vi "Test@ShowCMD__Parameter.vi"(1 "ParamterIn":string) -> (0 "ParamterOut":string)   [LabVIEW 2019]
panel:
  in  "Device":string(combo)
  in  "Confirm":bool
  # "Test@ShowCMD $ExternDevice"
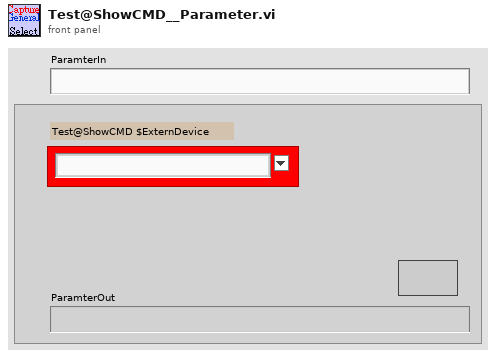
[diagram p1: front panel]
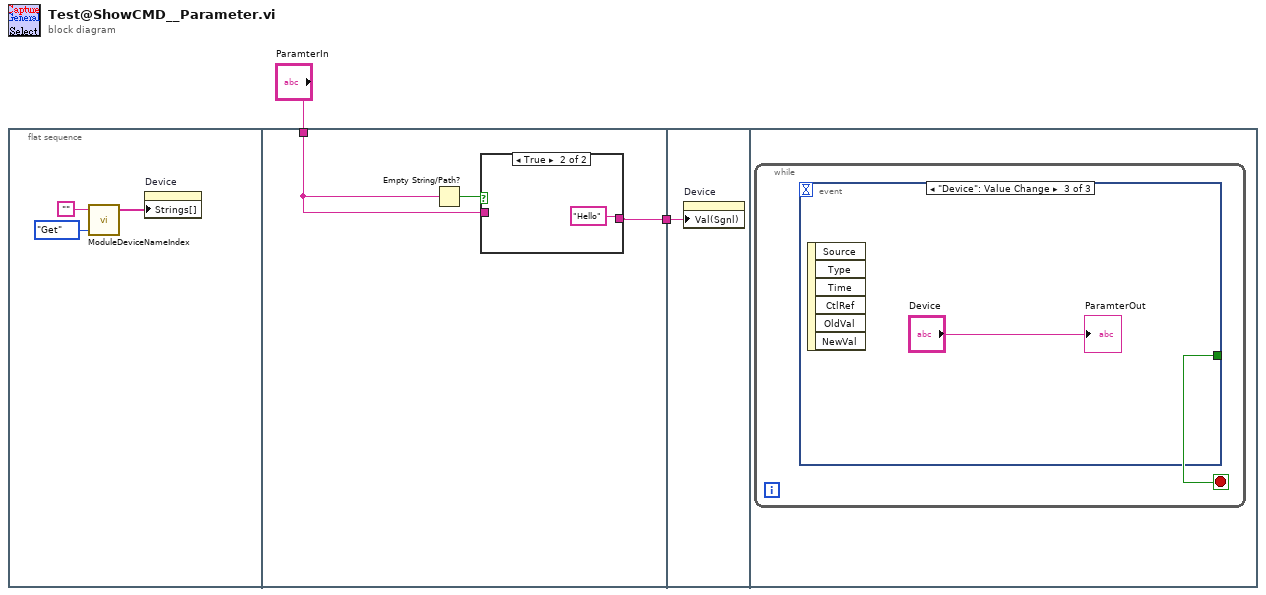
[diagram p0: block diagram]
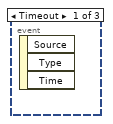
[diagram p3: hidden frame]
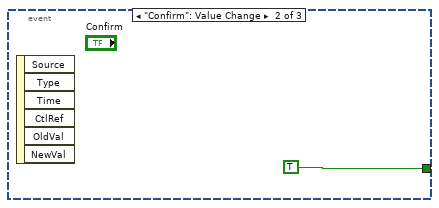
[diagram p4: hidden frame]
diagram:
  n1 = flat-sequence {
    tunnel: "ParamterIn" -> [w7]
    tunnel: [w6] -> w1
    tunnel: w1 -> [w11]
    frame #0 {
      n2 = call "ModuleDeviceNameIndex.vi"("OP"=enum16{"Get", "Update", "Init"}."Get", "DeviceName"="") -> ("DeviceList"=w4:string[])  [unwired: 1 in, 2 out]
      n3 = property on="Device" class="CmbBox"("Strings[]"=w4) -> ()  [unwired: 2 in, 2 out]
    }
    frame #1 {
      n4 = Empty String/Path?(string/path=w7) -> (empty?=w8:bool)
      n5 = case shown="True" w8 {
        tunnel: w7 -> [w9 _]
        tunnel: [w9 "Hello" ("ParamterIn")] -> w6
        frame False {
        }
        frame True {
        }
      }
    }
    frame #2 {
      n6 = property on="Device" class="CmbBox"("Val(Sgnl)"=w11) -> ()  [unwired: 2 in, 2 out]
    }
    frame #3 {
      n7 = while {
        stop <- w12 stop-if-true
        n8 = event shown="[2] \"Device\": Value Change" {
          selector: _ -> [_ _ _]
          dyn-events: _ -> [_ _ _]
          timeout: _ -> [_ _ _]
          tunnel: [_ TRUE _] -> w12
          event Timeout {
            n9 = event-data() -> ()  [unwired: 1 in, 3 out]
          }
          event "Confirm": Value Change {
            n10 = event-data() -> ()  [unwired: 1 in, 6 out]
          }
          event "Device": Value Change {
            n11 = event-data() -> ()  [unwired: 1 in, 6 out]
            "ParamterOut" <- "Device"
          }
        }
      }
    }
  }
